vi "test actor core.vi"(11 "Instr Actor in":refnum<class "Instr Actor.lvclass">) -> ()   [LabVIEW 2014, in "Instrument Library.lvlib" / "Instr Actor.lvclass"]
uses:
  Instr Actor.lvclass
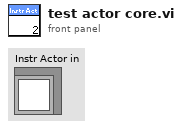
[diagram p1: front panel]
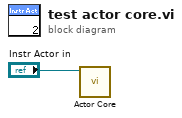
[diagram p0: block diagram]
diagram:
  n1 = call-dynamic "Actor Core.vi"("Instr Actor in"="Instr Actor in") -> ()  [unwired: 9 in, 2 out]
